vi "斐波拉契数列.vi"() -> ()   [LabVIEW 2017]
panel:
  out "Numeric 2":dbl
  in  "Numeric":dbl
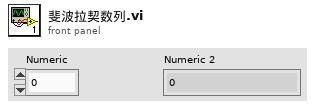
[diagram p1: front panel]
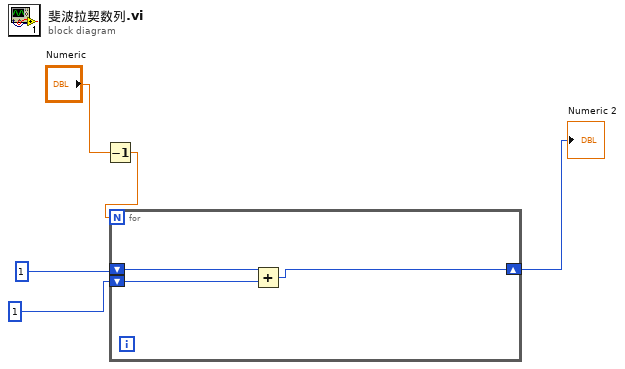
[diagram p0: block diagram]
diagram:
  n1 = Decrement(x="Numeric") -> (x-1=w1:dbl)
  n2 = for {
    N: w1 -> [_]
    shift-right: [w6] -> w3
    shift-left: 1 -> [w8]
    shift-left: 1 -> [w7]
    n3 = Add(x=w8, y=w7) -> (x+y=w6:i32)
  }
  "Numeric 2" <- w3
